vi "相机名称品牌启用状态.vi"() -> ()   [LabVIEW 2014]
uses:
  <vilib>/userdefined/High Color/IMAQdx.ctl
panel:
  in  "相机名称":T2={"相机1名称"="cam1", "相机2名称"="cam1", "相机3名称"="cam1", "相机4名称"="cam1", "Cam1启用"=FALSE, "Cam2启用"=FALSE, "Cam3启用"=FALSE, "Cam4启用"=FALSE, "Basler1"=FALSE, "Basler2"=FALSE, "Basler3"=FALSE, "Basler4"=FALSE}
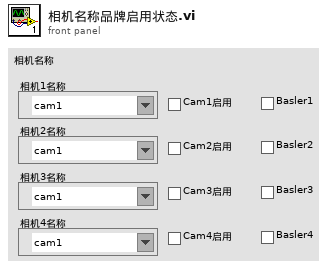
[diagram p1: front panel]
types:
  T1 = typedef "IMAQdx.ctl" = refnum<k21>
  T2 = cluster{"相机1名称":T1, "相机2名称":T1, "相机3名称":T1, "相机4名称":T1, "Cam1启用":bool, "Cam2启用":bool, "Cam3启用":bool, "Cam4启用":bool, "Basler1":bool, "Basler2":bool, "Basler3":bool, "Basler4":bool}
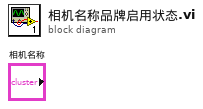
[diagram p0: block diagram]
diagram:
